vi "4155C Sample Config SMUs.vi"(4 "error in (no error)":errorcluster, 7 "VISA resource name in":refnum<visa-resource-name>) -> (0 "error out":errorcluster, 3 "VISA Resource Name out":refnum<visa-resource-name>)   [LabVIEW 2016]
panel:
  in  "Gate Standby":bool
  in  "Drain Standby":bool
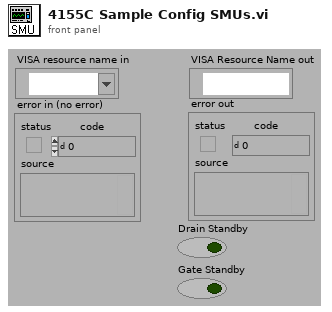
[diagram p1: front panel]
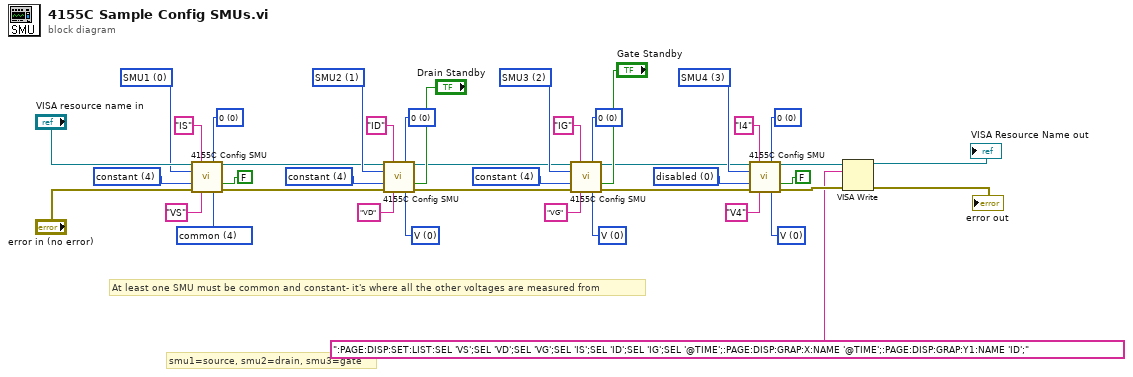
[diagram p0: block diagram]
diagram:
  w14 = u32 0 items=["V  ", "I  ", "V pulse  ", "I pulse  ", "  common  "] ("mode")
  w15 = u32 0 items=["0  ", "10K Ohms  ", "100K Ohms  ", "1M Ohms  "] ("series resistance *")
  w17 = u32 0 items=["disabled  ", "VAR1  ", "VAR2  ", "VAR1'  ", "constant  "] ("function")
  w18 = u32 3 items=["SMU1  ", "SMU2  ", "SMU3  ", "SMU4  ", "SMU5  ", "SMU6  "] ("unit to configure")
  w21 = u32 0 items=["V  ", "I  ", "V pulse  ", "I pulse  ", "  common  "] ("mode")
  w22 = u32 0 items=["0  ", "10K Ohms  ", "100K Ohms  ", "1M Ohms  "] ("series resistance *")
  w24 = u32 4 items=["disabled  ", "VAR1  ", "VAR2  ", "VAR1'  ", "constant  "] ("function")
  w25 = u32 2 items=["SMU1  ", "SMU2  ", "SMU3  ", "SMU4  ", "SMU5  ", "SMU6  "] ("unit to configure")
  w28 = u32 0 items=["V  ", "I  ", "V pulse  ", "I pulse  ", "  common  "] ("mode")
  w29 = u32 0 items=["0  ", "10K Ohms  ", "100K Ohms  ", "1M Ohms  "] ("series resistance *")
  w31 = u32 4 items=["disabled  ", "VAR1  ", "VAR2  ", "VAR1'  ", "constant  "] ("function")
  w32 = u32 1 items=["SMU1  ", "SMU2  ", "SMU3  ", "SMU4  ", "SMU5  ", "SMU6  "] ("unit to configure")
  w35 = u32 4 items=["V  ", "I  ", "V pulse  ", "I pulse  ", "  common  "] ("mode")
  w36 = u32 0 items=["0  ", "10K Ohms  ", "100K Ohms  ", "1M Ohms  "] ("series resistance *")
  w38 = u32 4 items=["disabled  ", "VAR1  ", "VAR2  ", "VAR1'  ", "constant  "] ("function")
  w39 = u32 0 items=["SMU1  ", "SMU2  ", "SMU3  ", "SMU4  ", "SMU5  ", "SMU6  "] ("unit to configure")
  # "smu1=source, smu2=drain, smu3=gate"
  # "At least one SMU must be common and constant- it's where all the other voltages are measured from"
  n1 = call "4155C Config SMU.vi"("VISA session"="VISA resource name in", "I name (max 6 chars)"="IS", "series resistance *"=w36, "unit to configure"=w39, "function"=w38, "standby"=FALSE, "error in (no error)"="error in (no error)", "V name (max 6 chars)"="VS", "mode"=w35) -> ("dup VISA resource name"=w11:refnum<visa-resource-name>, "error out"=w10:errorcluster)  [unwired: 5 in]
  n2 = call "4155C Config SMU.vi"("VISA session"=w11, "I name (max 6 chars)"="ID", "series resistance *"=w29, "unit to configure"=w32, "function"=w31, "standby"="Drain Standby", "error in (no error)"=w10, "V name (max 6 chars)"="VD", "mode"=w28) -> ("dup VISA resource name"=w8:refnum<visa-resource-name>, "error out"=w9:errorcluster)  [unwired: 5 in]
  n3 = call "4155C Config SMU.vi"("VISA session"=w8, "I name (max 6 chars)"="IG", "series resistance *"=w22, "unit to configure"=w25, "function"=w24, "standby"="Gate Standby", "error in (no error)"=w9, "V name (max 6 chars)"="VG", "mode"=w21) -> ("dup VISA resource name"=w7:refnum<visa-resource-name>, "error out"=w6:errorcluster)  [unwired: 5 in]
  n4 = call "4155C Config SMU.vi"("VISA session"=w7, "I name (max 6 chars)"="I4", "series resistance *"=w15, "unit to configure"=w18, "function"=w17, "standby"=FALSE, "error in (no error)"=w6, "V name (max 6 chars)"="V4", "mode"=w14) -> ("dup VISA resource name"=w5:refnum<visa-resource-name>, "error out"=w4:errorcluster)  [unwired: 5 in]
  n5 = VISA Write(VISA resource name=w5, write buffer=":PAGE:DISP:SET:LIST:SEL 'VS';SEL 'VD';SEL 'VG';SEL 'IS';SEL 'ID';SEL 'IG';SEL '@TIME';:PAGE:DISP:GRAP:X:NAME '@TIME';:PAGE:DISP:GRAP:Y1:NAME 'ID';" ("write buffer (\"\")"), error in (no error)=w4) -> (VISA resource name out=→"VISA Resource Name out":refnum<visa-resource-name>, error out=→"error out":errorcluster)  [unwired: 1 out]
